vi "Calculate refresh rate.vi"(11 "Frame size":u16) -> (0 "error out":errorcluster, 3 "Refresh rate (Hz)":i32 format="Frame Rate: %.0f fps")   [LabVIEW 2020]
uses:
  <userlib>/_MGI/Application Control/MGI Change Detector/MGI Change Detector (T).vi
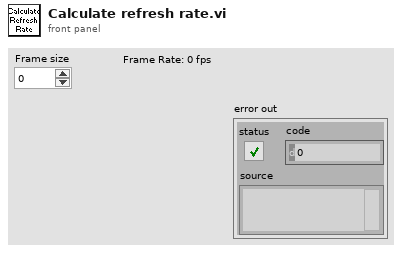
[diagram p1: front panel]
types:
  T1 = typedef "AOL_Globals.ctl" = cluster{"Imaging Protocol":T2, "Number of POI":u16, "Number of Miniscans":u16, "Number of Trials":u16, "Number of Cycles ":u64, "# Averaged Frames":u16, "Laser power (%)":u8, "Pockels (V)":dbl, "Acquisition Length (sec)":dbl, "Fill time (us)":dbl, "POI Dwell time (us)":dbl, "Miniscan Dwell time per pixel (us)":dbl, "PMT 1":dbl, "PMT 2":dbl, "Back Apperture (mA)":dbl, "Frame Size":T3, "Center Frequency":dbl, "Field of View (norm)":dbl, "DwellTime (us)":dbl, "Wavelength (nm)":dbl, "Zoom":dbl, "AOL Z":dbl, "AOL Mode":T4, "GridXY":dbl, "GridZ":dbl, "TriggerPeriod (sec)":dbl, "Number of Pixels in Miniscan":u16, "Experiment folder path":path, "X centre":dbl, "Y centre":dbl, "Angle (degrees)":dbl, "Plane Mode":T5, "Threshold":u16[], "Regenerate Chirps":bool, "Rectangle ROI length (pixels)":u16, "Rectangle ROI height (pixels)":u16, "AOD fill":u16, "StartupDelay":i32, "Samples Wait after Trigger":u16, "Slip Cycle":u32, "Add Cycle":bool, "Functional Mode":T6, "Z Start":dbl, "Z Stop":dbl, "# Planes":i32, "Total Pixels":i32, "Variable Miniscan Pixels":u16[], "Use Variable Length":bool, "Use Variable Resolution":bool, "Laser power (%) at Z Start":u8, "Laser power (%) at Z Stop":u8, "Ref Z Step":i8, "Ref Dwell Time (us)":dbl, "Field of View (um)":dbl}
  T2 = typedef "Imaging Protocols enum.ctl" = enum16{"AOL Z-Stack", "Motor Z Stack", "Functional Acquisition", "Single Plane Acquisition", "Volume Acquisition", "Live Imaging", "Live Plane Imaging", "Live Volume Imaging"}
  T3 = typedef "Frame Size.ctl" = u16
  T4 = typedef "AOL modes.ctl" = enum16{"Raster", "Structural", "Pointing", "Mini Scan", "Alignment"}
  T5 = typedef "Plane Mode.ctl" = u16
  T6 = typedef "Functional Mode.ctl" = enum16{"Point", "Line", "Patch", "Plane", "Volume"}
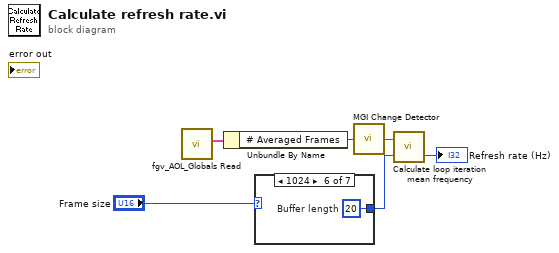
[diagram p0: block diagram]
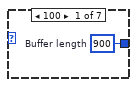
[diagram p2: hidden frame]
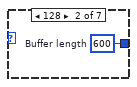
[diagram p3: hidden frame]
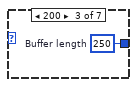
[diagram p4: hidden frame]
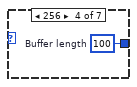
[diagram p5: hidden frame]
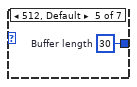
[diagram p6: hidden frame]
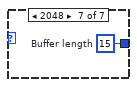
[diagram p7: hidden frame]
diagram:
  n1 = call "fgv_AOL_Globals Read.vi"() -> ("AOL_Globals"=w2:T1)  [unwired: 9 in, 2 out]
  n2 = Unbundle By Name(w2) -> ("# Averaged Frames"=w3:u16)
  n3 = case shown="1024" "Frame size" {
    tunnel: [w7 w8 w9 w10 w11 w12 w13] -> w5
    frame 100 {
      w7 = 900  # Buffer length
    }
    frame 128 {
      w8 = 600  # Buffer length
    }
    frame 200 {
      w9 = 250  # Buffer length
    }
    frame 256 {
      w10 = 100  # Buffer length
    }
    frame 512, Default {
      w11 = 30  # Buffer length
    }
    frame 1024 {
      w12 = 20  # Buffer length
    }
    frame 2048 {
      w13 = 15  # Buffer length
    }
  }
  n4 = call-poly <userlib>:"MGI Change Detector.vi"("Value"=w3) -> ("Changed?"=w4:bool)
  n5 = call "Calculate loop iteration mean frequency.vi"("Buffer length (10 points)"=w5, "Instant output during setup changes"=w4) -> ("Refresh rate (Hz)"=→"Refresh rate (Hz)":i32)  [unwired: 1 in]
